vi "Multiply Force.vi"(10 "force in":dbl, 11 "Prybar in":refnum<class "Prybar.lvclass">) -> (2 "force out":dbl)   [LabVIEW 2023, in "Prybar.lvclass"]
uses:
  Prybar.lvclass
  Prybar.lvclass/Prybar.ctl
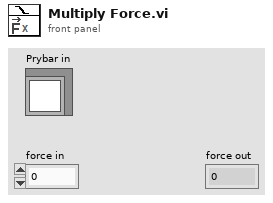
[diagram p1: front panel]
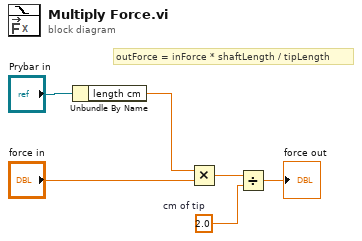
[diagram p0: block diagram]
diagram:
  w1 = 2.0  # cm of tip
  # "outForce = inForce * shaftLength / tipLength"
  n1 = Unbundle By Name("Prybar in") -> ("length cm"=w2:dbl)
  n2 = Multiply(x=w2, y="force in") -> (x*y=w4:dbl)
  n3 = Divide(x=w4, y=w1) -> (x/y=→"force out":dbl)
